vi "dxfinterpreter.vi"(8 "error in (no error)":errorcluster) -> (0 "error out":errorcluster, 1 "Geo":cluster{string, dbl[]}[](array[cluster]), 2 "name":string, 3 "stripped path":path)   [LabVIEW 2018]
panel:
  out "LineType":string[](array[string])
  # "Connector Pane"
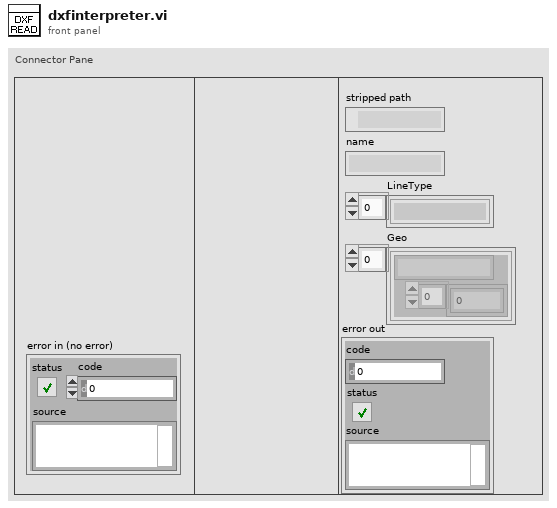
[diagram p1: front panel]
types:
  T1 = typedef "dxf typedef.lvlib/singleDXFobject.ctl" = cluster{"ID":T2, "Data":T2[]}
  T2 = typedef "dxf typedef.lvlib/singleDXFvar.ctl" = cluster{"GroupCode":string, "Value":string}
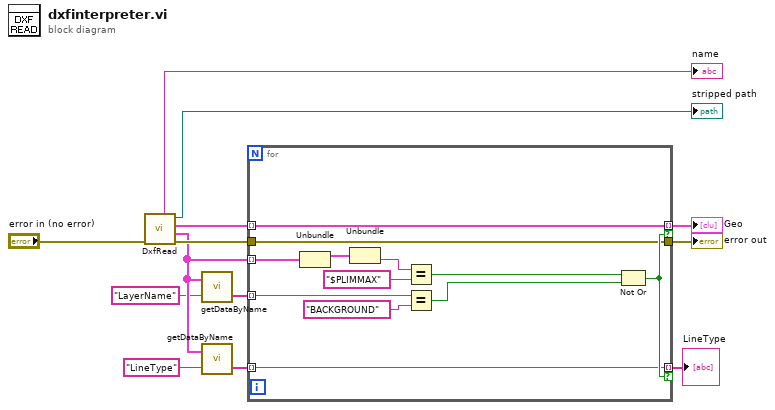
[diagram p0: block diagram]
diagram:
  n1 = call "DxfRead.vi"("error in (no error)"="error in (no error)") -> ("error out"=w12:errorcluster, "Array 2"=w4:T1[], "Array"=w8:cluster{string, dbl[]}[], "stripped path"=→"stripped path":path, "name"=→"name":string)  [unwired: 6 in]
  n2 = call "getDataByName.vi"("Data Entry Name"="LayerName" ("y"), "Property Array In"=w4) -> ("Value"=w7:string[])  [unwired: 1 out]
  n3 = call "getDataByName.vi"("Data Entry Name"="LineType", "Property Array In"=w4) -> ("Value"=w6:string[])  [unwired: 1 out]
  n4 = for {
    tunnel: w4 -> [w25] mode=indexing
    tunnel: w8 -> [w17] mode=indexing
    tunnel: w6 -> [w14] mode=indexing
    tunnel: w7 -> [w20] mode=indexing
    tunnel: [w17] -> w2 mode=indexing if=w16
    tunnel: [w14] -> w1 mode=indexing if=w16
    tunnel: [w15] -> w13
    tunnel: w12 -> [w15]
    n5 = Unbundle(w25) -> ("ID"=w24:T2)  [unwired: 1 out]
    n6 = Unbundle(w24) -> ("Value"=w23:string)  [unwired: 1 out]
    n7 = Equal?(x=w23, y="$PLIMMAX") -> (x = y?=w22:bool)
    n8 = Equal?(x=w20, y="BACKGROUND") -> (x = y?=w18:bool)
    n9 = Not Or(1:w18, 2:w22) -> (0:w16:bool)
  }
  "error out" <- w13
  "Geo" <- w2
  "LineType" <- w1
